vi "Check Internal.vi"(5 "Max Range":cluster{i64, i64, i64}, 6 "Points":cluster{i64, i64, i64}[](array[cluster]), 7 "Min Range":cluster{i64, i64, i64}, 11 "Point to Check":cluster{i64, i64, i64}) -> (3 "Internal?":bool=TRUE)   [LabVIEW 2021, in "d18.lvlib"]
uses:
  d18.lvlib
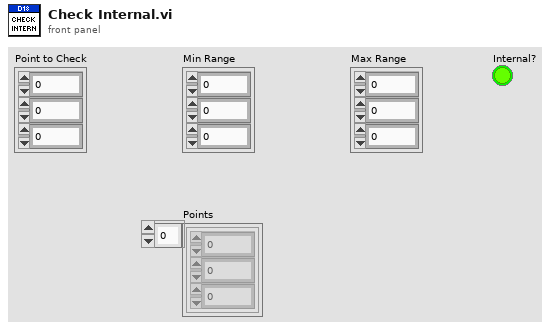
[diagram p1: front panel]
types:
  T1 = cluster{"key not found?":bool, cluster{"Set?":bool, "Internal?":bool}}
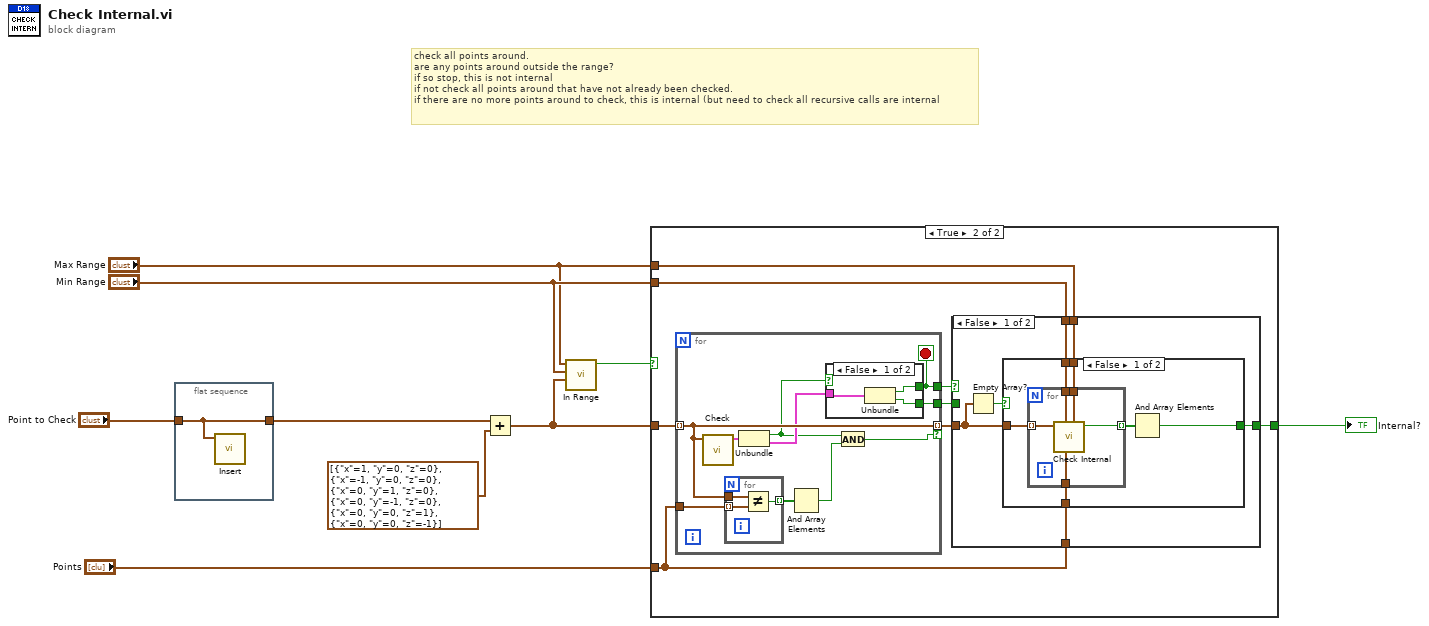
[diagram p0: block diagram]
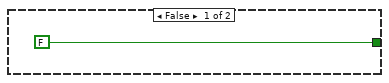
[diagram p2: hidden frame]
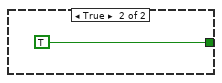
[diagram p3: hidden frame]
diagram:
  # "check all points around.\nare any points around outside the range?\nif so stop, this is not internal\nif not check all points around that have not already been checked.\nif there are no more points around to check, this is internal (but need to check all recursive calls are internal"
  n1 = flat-sequence {
    tunnel: "Point to Check" -> [w10]
    tunnel: [w10] -> w3
    frame #0 {
      n2 = call "Insert.vi"("point"=w10) -> ()  [unwired: 10 in, 1 out]
    }
  }
  n3 = Add(x=w3, y=cluster{"x":i64, "y":i64, "z":i64}[] [{"x"=1, "y"=0, "z"=0}, {"x"=-1, "y"=0, "z"=0}, {"x"=0, "y"=1, "z"=0}, {"x"=0, "y"=-1, "z"=0}, {"x"=0, "y"=0, "z"=1}, {"x"=0, "y"=0, "z"=-1}]) -> (x+y=w4:cluster{i64, i64, i64}[])
  n4 = call "In Range.vi"("Array"=w4, "Min Range"="Min Range", "Max Range"="Max Range") -> ("Boolean"=w6:bool)  [unwired: 8 in]
  n5 = case shown="True" w6 {
    tunnel: [FALSE ("Internal?") w17] -> w2
    tunnel: "Points" -> [_ w14]
    tunnel: "Min Range" -> [_ w19]
    tunnel: "Max Range" -> [_ w18]
    tunnel: w4 -> [_ w16]
    frame False {
    }
    frame True {
      n6 = for {
        tunnel: w16 -> [w46] mode=indexing
        tunnel: [w46] -> w15 mode=indexing if=w39
        tunnel: w14 -> [w47]
        tunnel: [w43] -> w13
        tunnel: [w42] -> w12
        stop <- w43 stop-if-true
        n7 = call "Check.vi"("Point to Check"=w46) -> ("response"=w48:T1)  [unwired: 10 in]
        n8 = for {
          tunnel: w47 -> [w54] mode=indexing
          tunnel: w46 -> [w53]
          tunnel: [w52] -> w45 mode=indexing
          n9 = Not Equal?(x=w53, y=w54) -> (x != y?=w52:bool)
        }
        n10 = Unbundle(w48) -> ("key not found?"=w41:bool, w44:cluster{"Set?":bool, "Internal?":bool})
        n11 = And Array Elements(Boolean array=w45) -> (logical AND=w40:bool)
        n12 = case shown="False" w41 {
          tunnel: w44 -> [w51 _]
          tunnel: [w50 _] -> w43
          tunnel: [w49 _] -> w42
          frame False {
            n13 = Unbundle(w51) -> ("Set?"=w50:bool, "Internal?"=w49:bool)
          }
          frame True {
          }
        }
        n14 = And(x=w41, y=w40) -> (x .and. y?=w39:bool)
      }
      n15 = case shown="False" w13 {
        tunnel: w19 -> [w25 _]
        tunnel: w18 -> [w24 _]
        tunnel: [w23 w38] -> w17
        tunnel: w15 -> [w21 _]
        tunnel: w14 -> [w20 _]
        tunnel: w12 -> [_ w38]
        frame False {
          n16 = Empty Array?(array=w21) -> (empty?=w22:bool)
          n17 = case shown="False" w22 {
            tunnel: w20 -> [w31 _]
            tunnel: w25 -> [w29 _]
            tunnel: w24 -> [w28 _]
            tunnel: [w26 TRUE] -> w23
            tunnel: w21 -> [w27 _]
            frame False {
              n18 = for {
                tunnel: w31 -> [w36]
                tunnel: w29 -> [w34]
                tunnel: w28 -> [w33]
                tunnel: w27 -> [w32] mode=indexing
                tunnel: [w35] -> w30 mode=indexing
                n19 = call "Check Internal.vi"("Max Range"=w33, "Points"=w36, "Min Range"=w34, "Point to Check"=w32) -> ("Internal?"=w35:bool)  [unwired: 7 in]
              }
              n20 = And Array Elements(Boolean array=w30) -> (logical AND=w26:bool)
            }
            frame True {
            }
          }
        }
        frame True {
        }
      }
    }
  }
  "Internal?" <- w2
